vi "XY Telemetry Output Test.vi"() -> ()   [LabVIEW 2017]
uses:
  Flow Control Enum.ctl
panel:
  out "new data from PC":bool
  out "XY Complete?":bool
  in  "stop":bool
  out "Y Acceleration":dbl(graph)
  out "Y Dispacement":dbl(graph)
  out "Y Speed PID":cluster{"Speed SP":dbl, "Speed PV":dbl}(graph)
  out "X Acceleration":dbl(graph)
  out "X Dispacement":dbl(graph)
  out "X Speed PID":cluster{"Speed SP":dbl, "Speed PV":dbl}(graph)
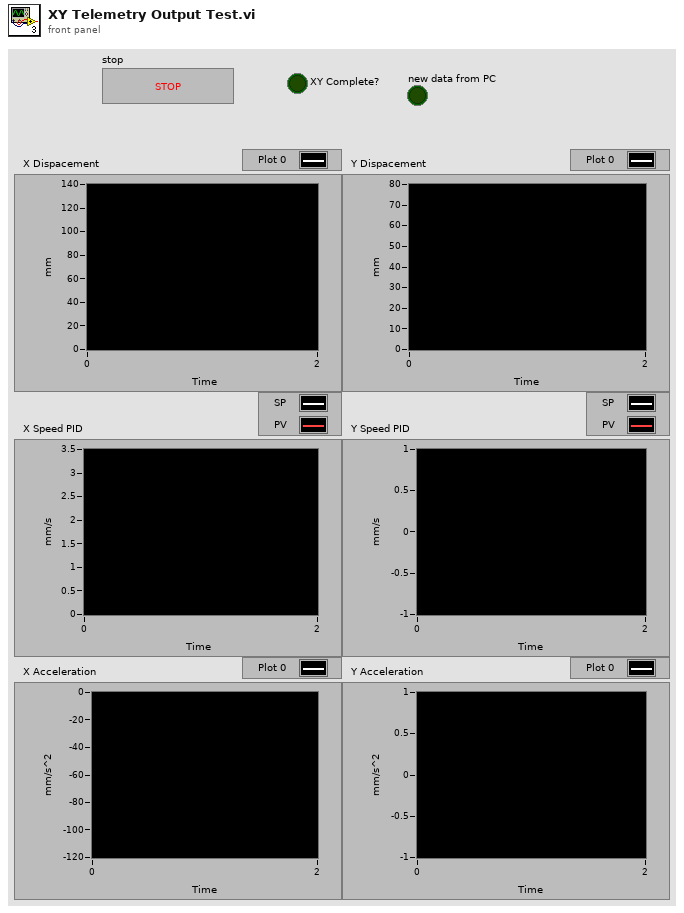
[diagram p1: front panel]
types:
  T1 = cluster{"X Coord":dbl, "Y Coord":dbl, "Energy":dbl, "Theta Angle":dbl}
  T2 = cluster{"X Coord":bool, "Y Coord":bool, "Energy":bool, "Theta Angle":bool}
  T3 = cluster{"X Axis":cluster{"Displacement":dbl, "Speed SP":dbl, "Speed PV":dbl, "Acceleration":dbl}, "Y Axis":cluster{"Displacement":dbl, "Speed SP":dbl, "Speed PV":dbl, "Acceleration":dbl}, "XY Complete?":bool}
  T4 = cluster{"Displacement":dbl, "Speed SP":dbl, "Speed PV":dbl, "Acceleration":dbl}
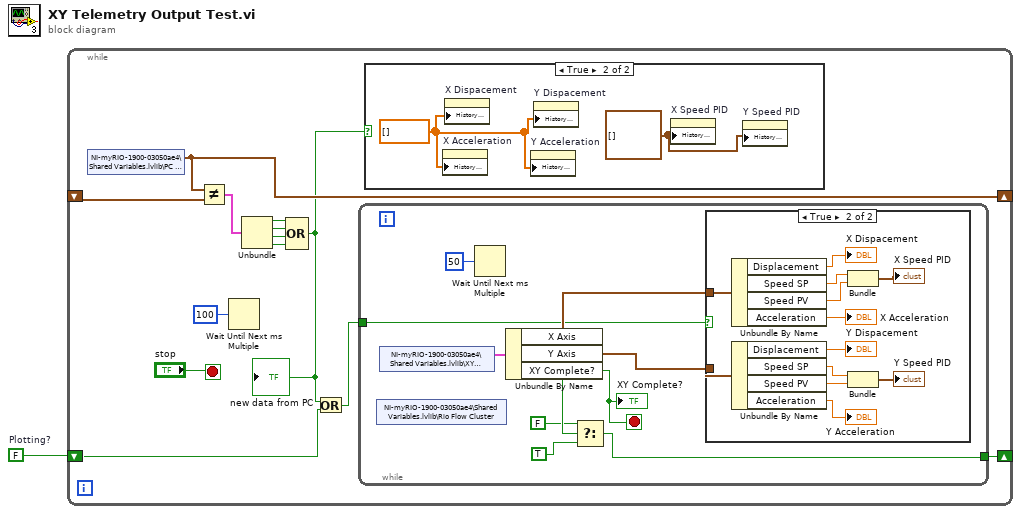
[diagram p0: block diagram]
diagram:
  w1 = FALSE  # Plotting?
  n1 = while {
    shift-right: [w12] -> _
    shift-left: _ -> [w13]
    shift-right: [w3] -> _
    shift-left: w1 -> [w5]
    stop <- "stop" stop-if-true
    n2 = shared-variable "NI-myRIO-1900-03050ae4\\Shared Variables.lvlib\\PC To Rio"() -> (w12:T1)  [unwired: 1 in, 1 out]
    n3 = Not Equal?(x=w12, y=w13) -> (x != y?=w11:T2)
    n4 = Wait Until Next ms Multiple(millisecond multiple=u32 100) -> ()  [unwired: 1 out]
    n5 = Unbundle(w11) -> ("X Coord"=w10:bool, "Y Coord"=w9:bool, "Energy"=w8:bool, "Theta Angle"=w7:bool)
    n6 = Compound Arithmetic op=OR(w10, w9, w8, w7) -> (w6:bool)
    "new data from PC" <- w6
    n7 = Or(x=w6, y=w5) -> (x .or. y?=w2:bool)
    n8 = while {
      tunnel: [w16] -> w3
      tunnel: w2 -> [w15]
      stop <- w19 stop-if-true
      n9 = shared-variable "NI-myRIO-1900-03050ae4\\Shared Variables.lvlib\\Rio Flow Cluster"() -> ()  [unwired: 1 in, 2 out]
      n10 = shared-variable "NI-myRIO-1900-03050ae4\\Shared Variables.lvlib\\XY Telemetry"() -> (w22:T3)  [unwired: 1 in, 1 out]
      n11 = Wait Until Next ms Multiple(millisecond multiple=u32 50) -> ()  [unwired: 1 out]
      n12 = Unbundle By Name(w22) -> ("X Axis"=w21:T4, "Y Axis"=w20:T4, "XY Complete?"=w19:bool)
      "XY Complete?" <- w19
      n13 = Select(t=FALSE, s=w19, f=TRUE) -> (s? t:f=w16:bool)
      n14 = case shown="True" w15 {
        tunnel: w21 -> [_ w25]
        tunnel: w20 -> [_ w24]
        frame False {
        }
        frame True {
          n15 = Unbundle By Name(w25) -> ("Displacement"=→"X Dispacement":dbl, "Speed SP"=w35:dbl, "Speed PV"=w34:dbl, "Acceleration"=→"X Acceleration":dbl)
          n16 = Unbundle By Name(w24) -> ("Displacement"=→"Y Dispacement":dbl, "Speed SP"=w29:dbl, "Speed PV"=w28:dbl, "Acceleration"=→"Y Acceleration":dbl)
          n17 = Bundle("Speed SP"=w35, "Speed PV"=w34) -> (→"X Speed PID":cluster{"Speed SP":dbl, "Speed PV":dbl})  [unwired: 1 in]
          n18 = Bundle("Speed SP"=w29, "Speed PV"=w28) -> (→"Y Speed PID":cluster{"Speed SP":dbl, "Speed PV":dbl})  [unwired: 1 in]
        }
      }
    }
    n19 = case shown="True" w6 {
      frame False {
      }
      frame True {
        w36 = cluster{"Speed SP":dbl, "Speed PV":dbl}[] [] ("History Data")
        w37 = dbl[] [] ("History Data")
        n20 = property on="X Acceleration" class="WFChart (strict)"("History Data"=w37) -> ()  [unwired: 2 in, 2 out]
        n21 = property on="X Dispacement" class="WFChart (strict)"("History Data"=w37) -> ()  [unwired: 2 in, 2 out]
        n22 = property on="Y Acceleration" class="WFChart (strict)"("History Data"=w37) -> ()  [unwired: 2 in, 2 out]
        n23 = property on="Y Dispacement" class="WFChart (strict)"("History Data"=w37) -> ()  [unwired: 2 in, 2 out]
        n24 = property on="X Speed PID" class="WFChart (strict)"("History Data"=w36) -> ()  [unwired: 2 in, 2 out]
        n25 = property on="Y Speed PID" class="WFChart (strict)"("History Data"=w36) -> ()  [unwired: 2 in, 2 out]
      }
    }
  }
